vi "Fluke Multimeter 3.vi"(8 "error in (no error)":errorcluster, 11 "Fluke Multimeter in":refnum<class "Fluke Multimeter.lvclass">) -> (0 "error out":errorcluster, 3 "Fluke Multimeter out":refnum<class "Fluke Multimeter.lvclass">)   [LabVIEW 2023, in "Fluke Multimeter.lvclass"]
uses:
  Fluke Multimeter.lvclass
  C:/LabVIEW-programs/Instruments/Utility Classes/Readable/Readable.lvclass
  Global/GPIB Numbers.vi
  Utility Classes/Readable/Readable.lvclass
panel:
  out "Status":string
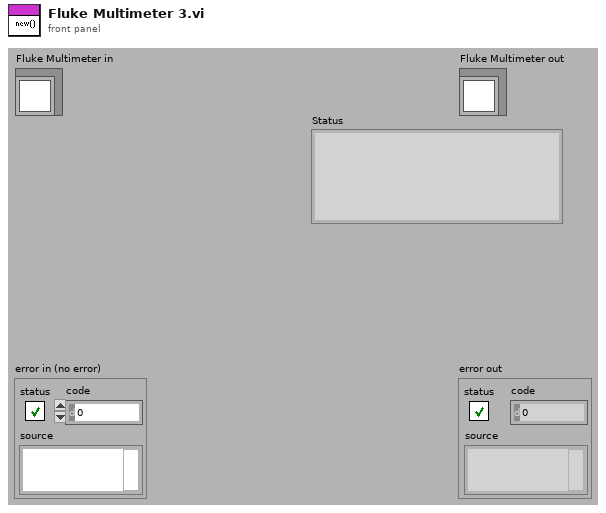
[diagram p1: front panel]
types:
  T1 = typedef "GPIB Type Def.ctl" = cluster{"Name":string, "bus":dbl, "GPIB":dbl, "GPIB as string":string, "byte":i32, "VISA Resource Name":refnum<visa-resource-name>}
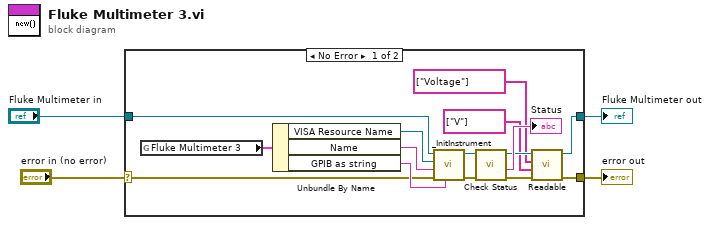
[diagram p0: block diagram]
diagram:
  n1 = case shown="No Error" "error in (no error)" {
    selector: "error in (no error)" -> [w12 w21]
    tunnel: [w10 w21] -> w3
    tunnel: [w7 w20] -> w1
    tunnel: "Fluke Multimeter in" -> [w17 w20]
    frame No Error {
      n2 = global read "GPIB Numbers.vi" "Fluke Multimeter 3"() -> (w19:T1)
      n3 = Unbundle By Name(w19) -> ("VISA Resource Name"=w16:refnum<visa-resource-name>, "Name"=w15:string, "GPIB as string"=w14:string)
      n4 = call-dynamic "_InitInstrument.vi"("GPIB as string"=w14, "error in (no error)"=w12, "Name"=w15, "VISA Resource Name"=w16, "Instrument in"=w17) -> ("error out"=w13:errorcluster, "Instrument out"=w18:refnum<class "Fluke Multimeter.lvclass">)  [unwired: 1 in, 4 out]
      n5 = call-dynamic "Check Status.vi"("error in (no error)"=w13, "Fluke Multimeter in"=w18) -> ("error out"=w9:errorcluster, "Status"=→"Status":string, "Fluke Multimeter out"=w8:refnum<class "Fluke Multimeter.lvclass">)  [unwired: 7 out]
      n6 = call "Readable.vi"("error in (no error)"=w9, "Channel Units"=string[] ["V"], "Channel Names"=string[] ["Voltage"], "Readable in"=w8) -> ("error out"=w10:errorcluster, "Readable out"=w7:refnum<class "Fluke Multimeter.lvclass">)  [unwired: 6 in]
    }
    frame Error {
    }
  }
  "error out" <- w3
  "Fluke Multimeter out" <- w1
